vi "CreateNiceXMLString.vi"(11 "XML In":string) -> (0 "XML String With IDs":string, 3 "XML String Human Readable":string)   [LabVIEW 2019]
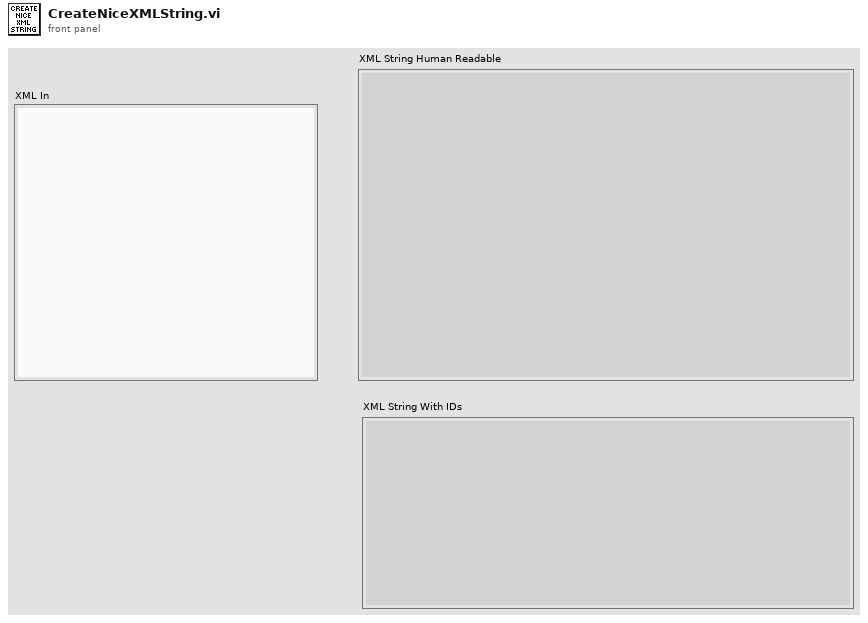
[diagram p1: front panel]
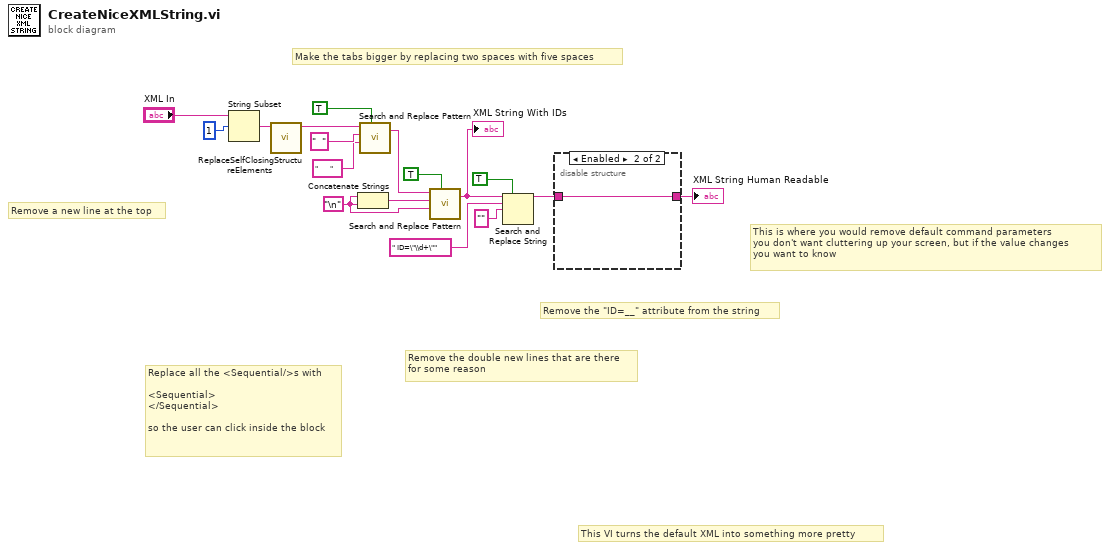
[diagram p0: block diagram]
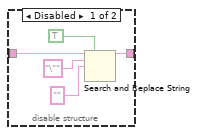
[diagram p2: hidden frame]
diagram:
  w14 = "\n"
  # "This is where you would remove default command parameters\nyou don't want cluttering up your screen, but if the value changes\nyou want to know"
  # "Remove the \"ID=__\" attribute from the string"
  # "Remove the double new lines that are there\nfor some reason"
  # "Make the tabs bigger by replacing two spaces with five spaces"
  # "Replace all the <Sequential/>s with\n\n<Sequential>\n</Sequential>\n\nso the user can click inside the block"
  # "Remove a new line at the top"
  # "This VI turns the default XML into something more pretty"
  n1 = String Subset(string="XML In", offset (0)=1) -> (substring=w8:string)  [unwired: 1 in]
  n2 = call "ReplaceSelfClosingStructureElements.vi"("String In"=w8) -> ("String Out"=w7:string)  [unwired: 10 in]
  n3 = Concatenate Strings(w14, w14) -> (w15:string)
  n4 = call <vilib>:"Search and Replace Pattern.vi"("string"=w7, "regular expression (\"\")"="  " ("regular expression (\"\")"), "replace string (\"\")"="      " ("regular expression (\"\")"), "replace all? (F)"=TRUE) -> ("result string"=w9:string)  [unwired: 1 in, 1 out]
  n5 = call <vilib>:"Search and Replace Pattern.vi"("string"=w9, "regular expression (\"\")"=w15, "replace string (\"\")"=w14, "replace all? (F)"=TRUE) -> ("result string"=w17:string)  [unwired: 1 in, 1 out]
  "XML String With IDs" <- w17
  n6 = Search and Replace String(replace all?=TRUE ("replace all? (F)"), input string=w17, search string=" ID=\"\\d+\"" ("format string"), replace string="" ("replace string (\"\")")) -> (result string=w2:string)  [unwired: 4 in, 3 out]
  n7 = disable-structure shown="Enabled" {
    disable-tunnel: w2 -> [w19 w23]
    disable-tunnel: [w18 w23] -> w1
    frame Disabled {
      n8 = Search and Replace String(replace all?=TRUE ("replace all? (F)"), input string=w19, search string="\"" ("format string"), replace string="" ("replace string (\"\")")) -> (result string=w18:string)  [unwired: 4 in, 3 out]
    }
    frame Enabled {
    }
  }
  "XML String Human Readable" <- w1
